vi "Generate INSERT SQL Query.vi"(8 "error in (no error)":errorcluster, 10 "Overlappping Records":refnum<class "Statement.lvclass">, 11 "Importing Transactions":refnum<class "Credit Statement.lvclass">) -> (0 "error out":errorcluster, 1 "Num records":i32, 3 "INSERT Query":string)   [LabVIEW 2018, in "Credit Statement.lvclass"]
uses:
  Credit Statement.lvclass
  Statement/Statement.lvclass
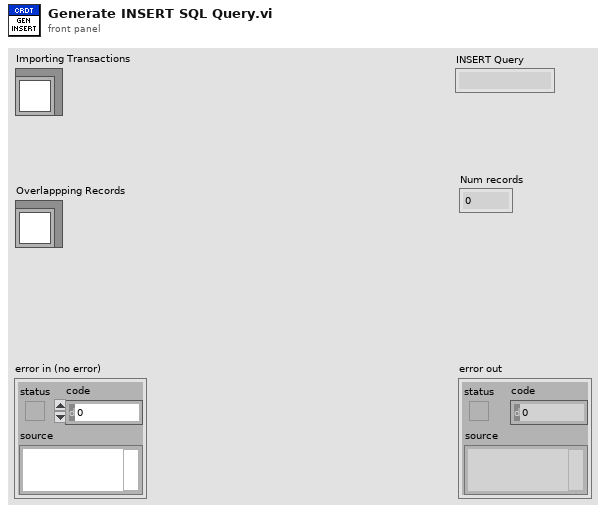
[diagram p1: front panel]
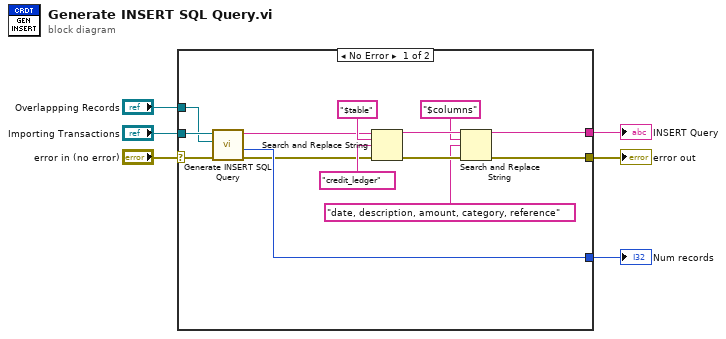
[diagram p0: block diagram]
diagram:
  n1 = case shown="No Error" "error in (no error)" {
    selector: "error in (no error)" -> [w9 w21]
    tunnel: [w20 _] -> w1
    tunnel: "Importing Transactions" -> [w19 _]
    tunnel: [w11 w21] -> w5
    tunnel: [w10 _] -> w4
    tunnel: "Overlappping Records" -> [w8 _]
    frame No Error {
      n2 = call-parent "Generate INSERT SQL Query.vi"("error in (no error)"=w9, "Overlappping Records"=w8, "Importing Transactions"=w19) -> ("error out"=w16:errorcluster, "Num records"=w20:i32, "INSERT Query"=w7:string)  [unwired: 6 in]
      n3 = Search and Replace String(input string=w7, search string="$table", replace string="credit_ledger" ("replace string (\"\")"), error in=w16) -> (result string=w14:string, error out=w15:errorcluster)  [unwired: 4 in, 2 out]
      n4 = Search and Replace String(input string=w14, search string="$columns", replace string="date, description, amount, category, reference", error in=w15) -> (result string=w10:string, error out=w11:errorcluster)  [unwired: 4 in, 2 out]
    }
    frame Error {
    }
  }
  "error out" <- w5
  "INSERT Query" <- w4
  "Num records" <- w1
